vi "series.vi"(1 "ic":dbl, 2 "m":dbl) -> (0 "s":dbl)   [LabVIEW 2023]
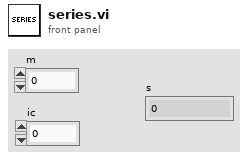
[diagram p1: front panel]
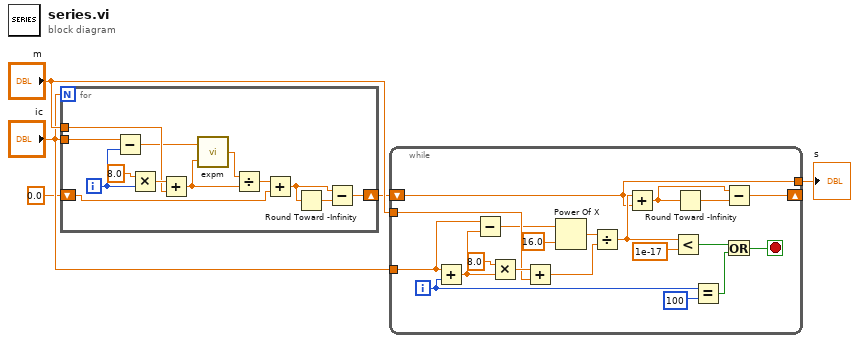
[diagram p0: block diagram]
diagram:
  n1 = for {
    N: "ic" -> [_]
    tunnel: "m" -> [w16]
    tunnel: "ic" -> [w15]
    shift-right: [w8] -> w2
    shift-left: 0.0 -> [w9]
    i -> [w14]
    n2 = Subtract(x=w15, y=w14) -> (x-y=w13:dbl)
    n3 = Multiply(x=8.0, y=w14) -> (x*y=w17:dbl)
    n4 = Add(x=w17, y=w16) -> (x+y=w11:dbl)
    n5 = call "expm.vi"("ak"=w11, "p"=w13) -> ("y"=w12:dbl)
    n6 = Divide(x=w12, y=w11) -> (x/y=w10:dbl)
    n7 = Add(x=w10, y=w9) -> (x+y=w6:dbl)
    n8 = Round Toward -Infinity(1:w6) -> (0:w7:dbl)
    n9 = Subtract(x=w6, y=w7) -> (x-y=w8:dbl)
  }
  n10 = while {
    tunnel: "ic" -> [w36]
    tunnel: "m" -> [w34]
    tunnel: [w22] -> w1
    shift-right: [w19] -> _
    shift-left: w2 -> [w22]
    i -> [w26]
    stop <- w27 stop-if-true
    n11 = Add(x=w36, y=w26) -> (x+y=w35:dbl)
    n12 = Subtract(x=w36, y=w35) -> (x-y=w31:dbl)
    n13 = Multiply(x=8.0, y=w35) -> (x*y=w38:dbl)
    n14 = Add(x=w38, y=w34) -> (x+y=w29:dbl)
    n15 = Power Of X(1:16.0 ("y"), 2:w31) -> (0:w30:dbl)
    n16 = Divide(x=w30, y=w29) -> (x/y=w28:dbl)
    n17 = Add(x=w28, y=w22) -> (x+y=w20:dbl)
    n18 = Less?(x=w28, y=1e-17) -> (x < y?=w23:bool)
    n19 = Round Toward -Infinity(1:w20) -> (0:w21:dbl)
    n20 = Equal?(x=w26, y=100) -> (x = y?=w24:bool)
    n21 = Subtract(x=w20, y=w21) -> (x-y=w19:dbl)
    n22 = Or(x=w23, y=w24) -> (x .or. y?=w27:bool)
  }
  "s" <- w1
